vi "AnalogOut_testing.vi"() -> ()   [LabVIEW 2013]
uses:
  <instrlib>/AnalogDiscSDKLv/VIs/DWF_Node.ctl
  <instrlib>/AnalogDiscSDKLv/VIs/DWF_Function.ctl
  <instrlib>/AnalogDiscSDKLv/AnalogDiscSDKLv.lvlib
  Windows/System32/dwf.dll
panel:
  out "error out":errorcluster
  out "error out2":errorcluster
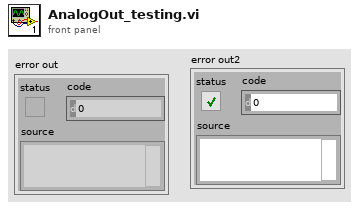
[diagram p1: front panel]
types:
  T1 = typedef "DWF_Node.ctl" = enum16{"Carrier", "FM", "AM"}
  T2 = typedef "DWF_Function.ctl" = u8
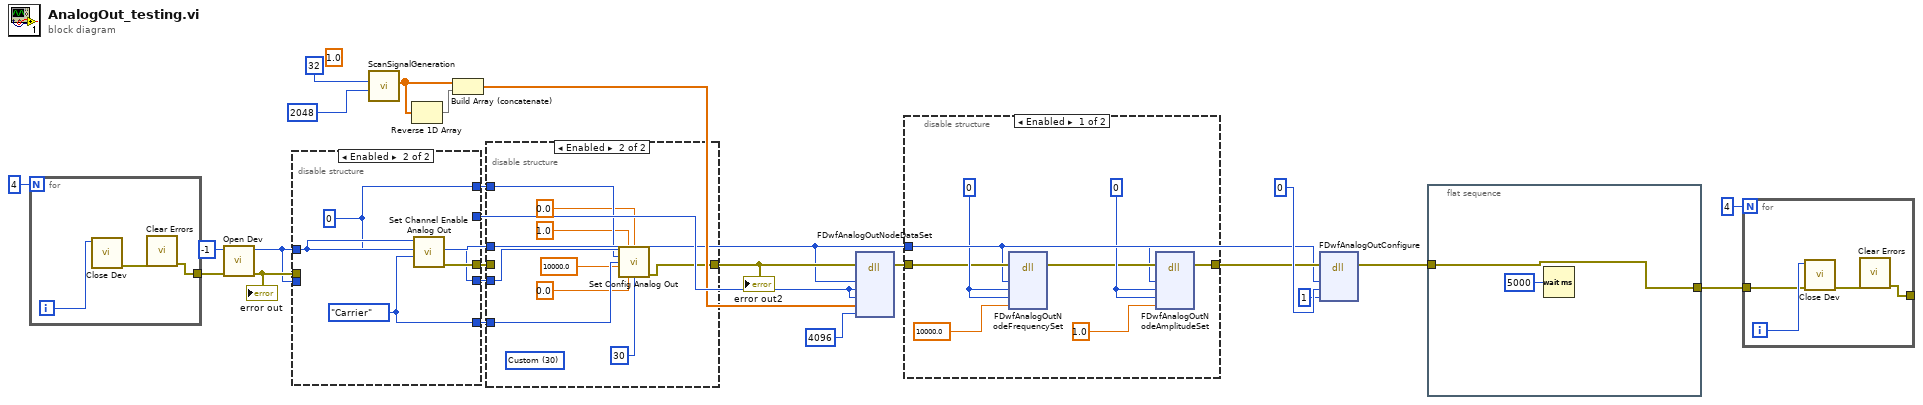
[diagram p0: block diagram]
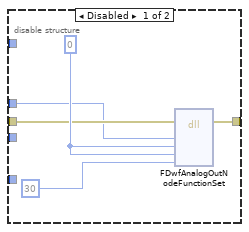
[diagram p3: hidden frame]
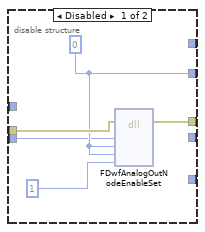
[diagram p4: hidden frame]
diagram:
  (unwired) 1.0 ("Amplitude")
  n1 = for {
    N: 4 -> [_]
    tunnel: [w25] -> w23
    i -> [w27]
    n2 = call <instrlib>:"Close Dev.vi"("hdwf"=w27) -> ("error out"=w26:errorcluster)  [unwired: 9 in, 1 out]
    n3 = call <vilib>:"Clear Errors.vi"("error in (no error)"=w26) -> ("error out"=w25:errorcluster)  [unwired: 6 in]
  }
  n4 = call <instrlib>:"Open Dev.vi"("error in (no error)"=w23, "idxDev"=-1) -> ("error out"=w22:errorcluster, "hdwf"=w5:i32)  [unwired: 7 in, 1 out]
  "error out" <- w22
  n5 = disable-structure shown="Enabled" {
    disable-tunnel: w22 -> [w32 _]
    disable-tunnel: [w30 _] -> w21
    disable-tunnel: [w29 w36] -> w14
    disable-tunnel: w5 -> [w28 _]
    disable-tunnel: w5 -> [_ w35]
    disable-tunnel: [_ w35] -> w4
    disable-tunnel: [_ w34] -> w3
    disable-tunnel: [_ w33] -> w2
    frame Disabled {
      w30 = 0
      n6 = dll-call lib="C:/Windows/System32/dwf.dll" fn="FDwfAnalogOutNodeEnableSet"(error in=w32, "h"=w28, "ch"=w30, "carrier"=w30, "fenable"=1) -> (error out=w29:errorcluster)  [unwired: 7 in, 1 out]
    }
    frame Enabled {
      w33 = DWF_Node."Carrier" ("node")
      w34 = 0 ("idxChannel")
      n7 = call <instrlib>:"Set Channel Enable Analog Out.vi"("node"=w33, "idxChannel"=w34, "hdwf"=w35) -> ("error out"=w36:errorcluster)  [unwired: 8 in]
    }
  }
  n8 = call "ScanSignalGeneration.vi"("NumRampPoints"=32, "NumPoints"=2048) -> ("Waveform"=w17:dbl[])  [unwired: 8 in, 1 out]
  n9 = Reverse 1D Array(array=w17) -> (reversed array=w18:dbl[])
  n10 = Build Array (concatenate)(w17, w18) -> (w16:dbl[])
  n11 = disable-structure shown="Enabled" {
    disable-tunnel: w14 -> [w39 _]
    disable-tunnel: [w38 w45] -> w13
    disable-tunnel: w5 -> [w37 _]
    disable-tunnel: w4 -> [_ w50]
    disable-tunnel: w3 -> [_ w49]
    disable-tunnel: w2 -> [_ w48]
    frame Disabled {
      w41 = 0
      n12 = dll-call lib="C:/Windows/System32/dwf.dll" fn="FDwfAnalogOutNodeFunctionSet"(error in=w39, "h"=w37, "ch"=w41, "carrier"=w41, "fenable"=30) -> (error out=w38:errorcluster)  [unwired: 7 in, 1 out]
    }
    frame Enabled {
      (unwired) T2 30 items=["DC"=0, "Sine"=1, "Square"=2, "Triangle"=3, "RampUp"=4, "RampDown"=5, "Noise"=6, "Custom"=30, "Play"=31] ("func")
      n13 = call <instrlib>:"Set Config Analog Out.vi"("hdwf"=w50, "vAmplitude"=1.0, "degPhase"=0.0, "idxChannel"=w49, "node"=w48, "hzFrequency"=10000.0, "vOffset"=0.0, "func"=30) -> ("error out"=w45:errorcluster)  [unwired: 6 in, 1 out]
    }
  }
  "error out2" <- w13
  n14 = dll-call lib="C:/Windows/System32/dwf.dll" fn="FDwfAnalogOutNodeDataSet"(error in=w13, "h"=w5, "ch"=w21, "carrier"=w21, "sample"=w16, "cdata"=4096) -> (error out=w11:errorcluster)  [unwired: 8 in, 1 out]
  n15 = disable-structure shown="Enabled" {
    disable-tunnel: w11 -> [w54 w59]
    disable-tunnel: [w52 w59] -> w10
    disable-tunnel: w5 -> [w51 _]
    frame Enabled {
      w56 = 0
      w57 = 0
      n16 = dll-call lib="C:/Windows/System32/dwf.dll" fn="FDwfAnalogOutNodeFrequencySet"(error in=w54, "h"=w51, "ch"=w57, "carrier"=w57, "freq"=10000.0) -> (error out=w53:errorcluster)  [unwired: 7 in, 1 out]
      n17 = dll-call lib="C:/Windows/System32/dwf.dll" fn="FDwfAnalogOutNodeAmplitudeSet"(error in=w53, "h"=w51, "ch"=w56, "carrier"=w56, "fenable"=1.0) -> (error out=w52:errorcluster)  [unwired: 7 in, 1 out]
    }
    frame Disabled {
    }
  }
  n18 = dll-call lib="C:/Windows/System32/dwf.dll" fn="FDwfAnalogOutConfigure"(error in=w10, "h"=w5, "ch"=0, "fstart"=1 ("carrier")) -> (error out=w8:errorcluster)  [unwired: 6 in, 1 out]
  n19 = flat-sequence {
    tunnel: w8 -> [w60]
    tunnel: [w60] -> w7
    frame #0 {
      n20 = Wait (ms)(milliseconds to wait=u32 5000) -> ()  [unwired: 1 out]
    }
  }
  n21 = for {
    N: 4 -> [_]
    tunnel: [w63] -> _
    tunnel: w7 -> [w62]
    i -> [w65]
    n22 = call <instrlib>:"Close Dev.vi"("error in (no error)"=w62, "hdwf"=w65) -> ("error out"=w64:errorcluster)  [unwired: 8 in, 1 out]
    n23 = call <vilib>:"Clear Errors.vi"("error in (no error)"=w64) -> ("error out"=w63:errorcluster)  [unwired: 6 in]
  }
